vi "parameter to Path_lvcicd.vi"(1 "String":string) -> (0 "Path":path)   [LabVIEW 2014, in "_lvcicd_support.lvlib"]
uses:
  _lvcicd_support.lvlib
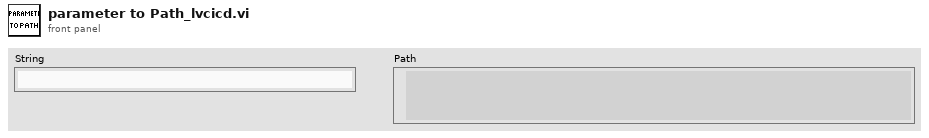
[diagram p1: front panel]
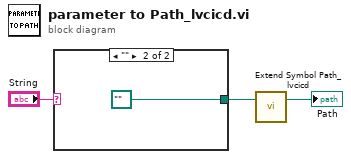
[diagram p0: block diagram]
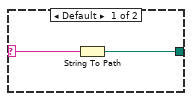
[diagram p2: hidden frame]
diagram:
  n1 = case shown="\"\"" "String" {
    selector: "String" -> [w5 _]
    tunnel: [w4 path ""] -> w2
    frame Default {
      n2 = String To Path(string=w5) -> (path=w4:path)
    }
    frame "" {
    }
  }
  n3 = call "Extend Symbol Path_lvcicd.vi"("Symbol Path"=w2) -> ("Resolved Path"=→"Path":path)  [unwired: 2 in]
